vi "RW_RS-485.vi"(8 "error in (no error)":errorcluster, 10 "Initial Command":string, 11 "VISA Refnum in":refnum<visa-resource-name>) -> (0 "error out":errorcluster, 2 "read buffer":string)   [LabVIEW 2018]
uses:
  <vilib>/Instr/_visa.llb/VISA Flush IO Buffer Mask.ctl
  <vilib>/Instr/_visa.llb/VISA Configure Serial Port (Instr).vi
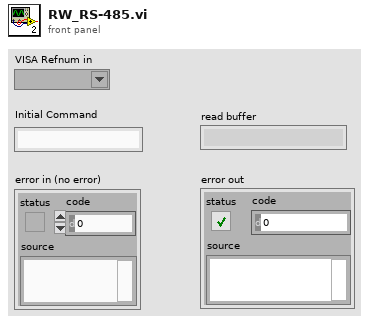
[diagram p1: front panel]
types:
  T1 = typedef "VISA Flush IO Buffer Mask.ctl" = u16
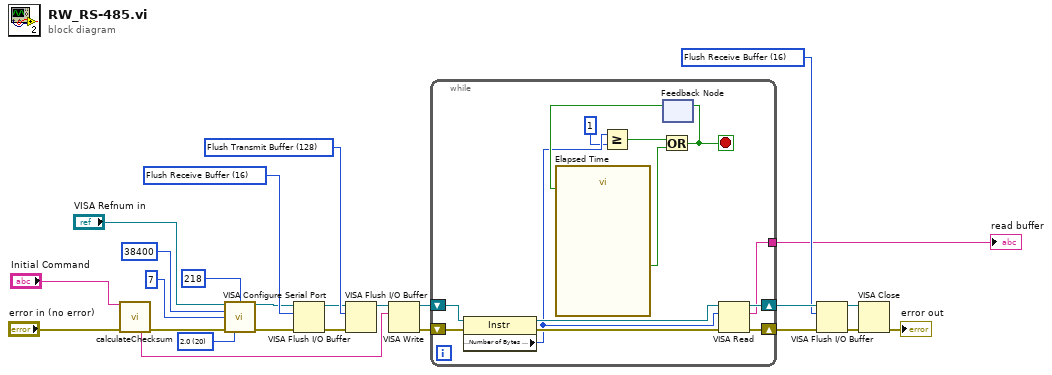
[diagram p0: block diagram]
diagram:
  w25 = u16 20 items=["1.0"=10, "1.5"=15, "2.0"=20] ("stop bits (10: 1 bit)")
  w14 = T1 128 items=["Flush Receive Buffer"=16, "Write Transmit Buffer to Device"=32, "Flush Receive Buffer (No I/O)"=64, "Flush Transmit Buffer"=128] ("Mask")
  w10 = T1 16 items=["Flush Receive Buffer"=16, "Write Transmit Buffer to Device"=32, "Flush Receive Buffer (No I/O)"=64, "Flush Transmit Buffer"=128] ("Mask")
  w7 = T1 16 items=["Flush Receive Buffer"=16, "Write Transmit Buffer to Device"=32, "Flush Receive Buffer (No I/O)"=64, "Flush Transmit Buffer"=128] ("Mask")
  n1 = call "calculateChecksum.vi"("Initial Command"="Initial Command", "error in (no error)"="error in (no error)") -> ("Start bit + Command + Check Sum + 2 Stop bits"=w20:string, "error out"=w21:errorcluster)  [unwired: 5 in, 7 out]
  n2 = call-poly "VISA Configure Serial Port"("VISA resource name"="VISA Refnum in", "termination char\n(0xA = '\\n' = LF)"=u8 218 ("termination char\n(0xA = '\\n' = LF)"), "baud rate (9600)"=u32 38400, "data bits (8)"=u16 7, "error in (no error)"=w21, "stop bits (10: 1 bit)"=w25) -> ("VISA resource name out"=w8:refnum<visa-resource-name>, "error out"=w9:errorcluster)  [unwired: 8 in]
  n3 = VISA Flush I/O Buffer(VISA resource name=w8, mask (16)=w10, error in (no error)=w9) -> (VISA resource name out=w13:refnum<visa-resource-name>, error out=w12:errorcluster)
  n4 = VISA Flush I/O Buffer(VISA resource name=w13, mask (16)=w14, error in (no error)=w12) -> (VISA resource name out=w15:refnum<visa-resource-name>)  [unwired: 1 out]
  n5 = VISA Write(VISA resource name=w15, write buffer=w20) -> (VISA resource name out=w4:refnum<visa-resource-name>, error out=w5:errorcluster)  [unwired: 1 in, 1 out]
  n6 = while {
    shift-right: [w33] -> w11
    shift-left: w4 -> [w38]
    shift-right: [w34] -> w6
    shift-left: w5 -> [w37]
    tunnel: [w28] -> w1
    stop <- w30 stop-if-true
    n7 = property class="Instr"(reference=w38, error in=w37) -> (reference out=w35:refnum<visa-resource-name>, error out=w36:errorcluster, "Serial Settings:Number of Bytes at Serial Port"=w27:u32)
    n8 = Greater Or Equal?(x=w27, y=u32 1 ("x")) -> (x >= y?=w32:bool)
    n9 = feedback #1() -> (w29:bool)  [unwired: 1 in]
    n10 = call "Elapsed Time"("Reset"=w29) -> ("Time has Elapsed"=w31:bool)  [unwired: 11 in, 7 out]
    n11 = Or(x=w32, y=w31) -> (x .or. y?=w30:bool)
    n12 = feedback-in #1(w30) -> ()
    n13 = VISA Read(VISA resource name=w35, byte count=w27, error in (no error)=w36) -> (VISA resource name out=w33:refnum<visa-resource-name>, read buffer=w28:string, error out=w34:errorcluster)  [unwired: 1 out]
  }
  "read buffer" <- w1
  n14 = VISA Flush I/O Buffer(VISA resource name=w11, mask (16)=w7, error in (no error)=w6) -> (VISA resource name out=w16:refnum<visa-resource-name>, error out=w17:errorcluster)
  n15 = VISA Close(VISA resource name=w16, error in (no error)=w17) -> (error out=→"error out":errorcluster)
